vi "Patrick-UTiLIA-Sim-Aq.vi"(4 "Cluster":T1={"1/f vs. Uniform "=1.0, "DC Drift Fraction"=0.0, "DC Drift Freq"=0.19999999999999996, "DC Offset"=0.0, "60Hz Amplitude"=0.001, "Gauss/Unif %"=0.5, "Sig Amp"=3.0, "Noise Amp"=0.001} {"Noise Amp" format="%.1p"; "Sig Amp" format="%.2p"; "Gauss/Unif %" min=0.0 max=1.0 step=0.05 format="%.2f"; "60Hz Amplitude" min=0.0 max=10.0 step=0.05 format="%.2p"; "DC Offset" min=-1.0 max=1.0 step=0.01 format="%.2f"; "DC Drift Freq" min=0.0 max=5.0 step=0.05 format="%.2f"; "DC Drift Fraction" format="%.2f"; "1/f vs. Uniform" min=0.0 max=50.0 step=0.5 format="%.1p"}, 5 "Sampling Info":cluster{"Fs":dbl[unit], "#S":i32}={"Fs"=71808.0, "#S"=16384}, 6 "Scaled Reference":dbl[](array[numeric])=array[16384 elements] format="%.2f", 7 "Error in":errorcluster) -> (0 "Applied Voltage":dbl[](array[numeric]) format="%.2f", 1 "Sample Voltage":dbl[](array[numeric]) format="%.2f", 3 "Error out":errorcluster)   [LabVIEW 2013]
uses:
  <vilib>/Analysis/2dsp.llb/Real FFT.vi
  <vilib>/Analysis/2dsp.llb/Inverse Real FFT.vi
  <vilib>/Analysis/3filter.llb/Butterworth Filter (DBL).vi
  <vilib>/measure/NI_MABase.lvlib
  <vilib>/Analysis/NI_AALPro.lvlib
  <vilib>/Analysis/NI_AALBase.lvlib
panel:
  out "Added Noise":dbl[](array[numeric]) format="%.2f"
  out "Waveforms":dbl[][](graph)
  # "Pass Through DAQ Info"
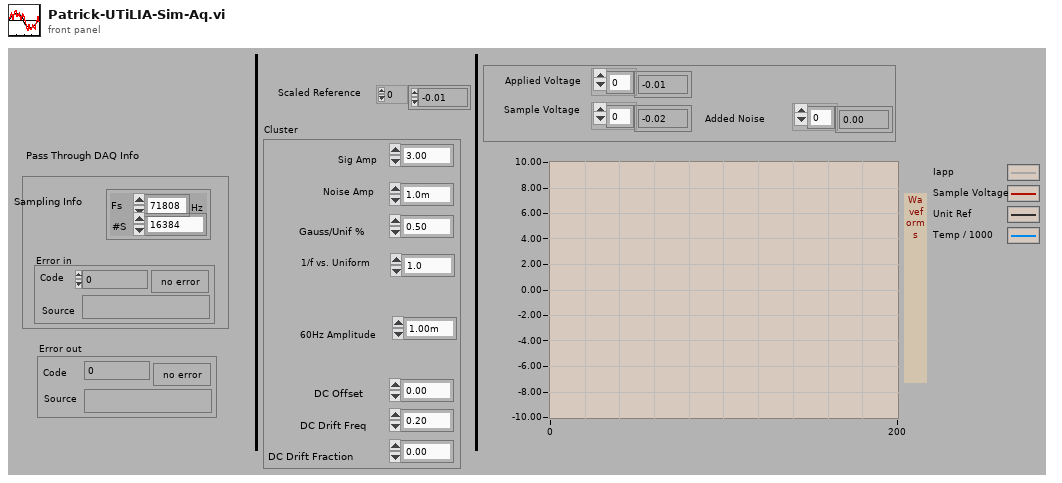
[diagram p1: front panel]
types:
  T1 = cluster{"1/f vs. Uniform ":dbl, "DC Drift Fraction":dbl, "DC Drift Freq":dbl, "DC Offset":dbl, "60Hz Amplitude":dbl, "Gauss/Unif %":dbl, "Sig Amp":dbl, "Noise Amp":dbl}
  T2 = enum32{"Lowpass", "Highpass", "Bandpass", "Bandstop"}
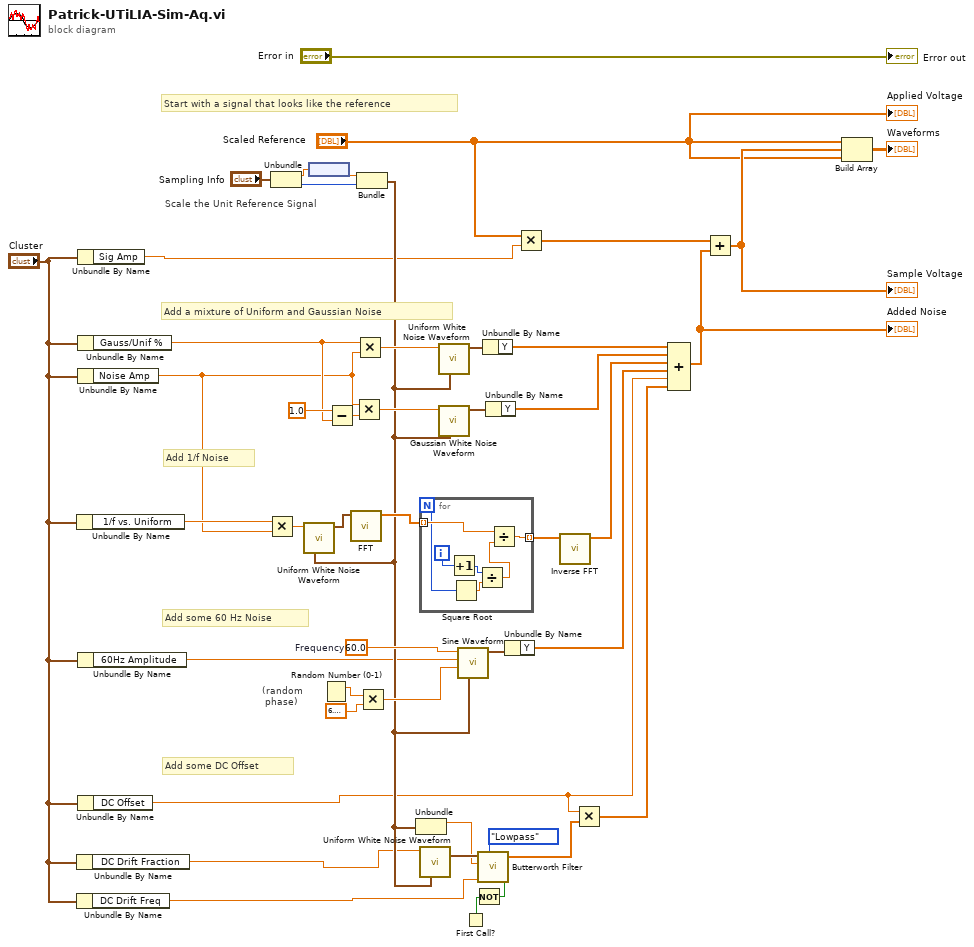
[diagram p0: block diagram]
diagram:
  w39 = 60.0  # Frequency
  # "Start with a signal that looks like the reference"
  # "Add 1/f Noise"
  # "(random\n phase)"
  # "Scale the Unit Reference Signal"
  # "Add some DC Offset"
  # "Add some 60 Hz Noise"
  # "Add a mixture of Uniform and Gaussian Noise"
  n1 = Unbundle By Name("Cluster") -> ("1/f vs. Uniform"=w7:dbl)
  n2 = Unbundle By Name("Cluster") -> ("DC Drift Fraction"=w1:dbl)
  n3 = Unbundle By Name("Cluster") -> ("DC Drift Freq"=w2:dbl)
  n4 = Unbundle By Name("Cluster") -> ("Sig Amp"=w9:dbl)
  n5 = Unbundle By Name("Cluster") -> ("Gauss/Unif %"=w8:dbl)
  n6 = Unbundle By Name("Cluster") -> ("Noise Amp"=w6:dbl)
  n7 = Unbundle By Name("Cluster") -> ("60Hz Amplitude"=w5:dbl)
  n8 = Unbundle By Name("Cluster") -> ("DC Offset"=w4:dbl)
  n9 = Multiply(x=w7, y=w6) -> (x*y=w25:dbl)
  n10 = Unbundle("Sampling Info") -> ("Fs"=w16:dbl[unit], "#S"=w17:i32)
  n11 = node(w16) -> (w20:dbl)
  n12 = Random Number (0-1)() -> (number: 0 to 1=w37:dbl)
  n13 = Subtract(x=1.0, y=w8) -> (x-y=w41:dbl)
  n14 = Multiply(x=w6, y=w41) -> (x*y=w43:dbl)
  n15 = Multiply(x=w8, y=w6) -> (x*y=w42:dbl)
  n16 = Bundle(w20, "#S"=w17) -> (w18:cluster{dbl, "#S":i32})  [unwired: 1 in]
  n17 = call <vilib>:"Uniform White Noise Waveform.vi"("sampling info"=w18, "amplitude"=w25) -> ("signal out"=w24:waveform(dbl))  [unwired: 8 in, 1 out]
  n18 = call-poly <vilib>:"FFT.vi"("X"=w24) -> ("FFT {X}"=w27:cdb[])  [unwired: 9 in, 1 out]
  n19 = Multiply(x=w37, y=6.283185307179586) -> (x*y=w36:dbl)
  n20 = Unbundle(w18) -> (w33:dbl)  [unwired: 1 out]
  n21 = for {
    N -> [w50]
    tunnel: [w53] -> w26 mode=indexing
    tunnel: w27 -> [w52] mode=indexing
    i -> [w51]
    n22 = Increment(x=w51) -> (x+1=w48:i32)
    n23 = Square Root(x=w50) -> (sqrt(x)=w49:dbl)
    n24 = Divide(x=w48, y=w49) -> (x/y=w47:dbl)
    n25 = Divide(x=w52, y=w47) -> (x/y=w53:cdb)
  }
  n26 = call <vilib>:"Uniform White Noise Waveform.vi"("sampling info"=w18, "amplitude"=w1) -> ("signal out"=w34:waveform(dbl))  [unwired: 8 in, 1 out]
  n27 = call <vilib>:"Uniform White Noise Waveform.vi"("sampling info"=w18, "amplitude"=w42) -> ("signal out"=w44:waveform(dbl))  [unwired: 8 in, 1 out]
  n28 = call <vilib>:"Gaussian White Noise Waveform.vi"("sampling info"=w18, "standard deviation"=w43) -> ("signal out"=w45:waveform(dbl))  [unwired: 8 in, 1 out]
  n29 = call <vilib>:"Sine Waveform.vi"("sampling info"=w18, "phase"=w36, "amplitude"=w5, "frequency"=w39) -> ("signal out"=w35:waveform(dbl))  [unwired: 6 in, 1 out]
  n30 = First Call?() -> (First Call?: T/F=w10:bool)
  n31 = Not(x=w10) -> (.not. x?=w31:bool)
  n32 = call-poly <vilib>:"Butterworth Filter.vi"("init/cont (init:F)"=w31, "filter type"=T2."Lowpass", "low cutoff freq: fl"=w2, "sampling freq: fs"=w33, "X"=w34) -> ("Filtered X"=w30:dbl[])  [unwired: 3 in, 1 out]
  n33 = Unbundle By Name(w44) -> ("Y"=w28:dbl[])
  n34 = Unbundle By Name(w45) -> ("Y"=w11:dbl[])
  n35 = Unbundle By Name(w35) -> ("Y"=w23:dbl[])
  n36 = Multiply(x="Scaled Reference", y=w9) -> (x*y=w29:dbl[])
  n37 = call-poly <vilib>:"Inverse FFT.vi"("FFT {X}"=w26) -> ("X"=w22:dbl[])  [unwired: 9 in, 1 out]
  n38 = Multiply(x=w4, y=w30) -> (x*y=w21:dbl[])
  n39 = Compound Arithmetic op=ADD(w28, w11, w22, w23, w4, w21) -> (w14:dbl[])
  "Added Noise" <- w14
  n40 = Add(x=w29, y=w14) -> (x+y=w13:dbl[])
  "Sample Voltage" <- w13
  n41 = Build Array("Scaled Reference", w13, "Scaled Reference") -> (→"Waveforms":dbl[][])
  "Error out" <- "Error in"
  "Applied Voltage" <- "Scaled Reference"
